vi "ConnectTestDisconnect.vi"() -> ()   [LabVIEW 2019]
panel:
  in  "CircleCenterFinder":bool
  in  "Circle Descriptor":cluster{"Min Radius":dbl, "Max Radius":dbl}={"Min Radius"=50.0, "Max Radius"=80.0}
  out "CircleCenterGH(mm)":string
  out "Image":T1(plugin-control)
  out "NumCirclesFound":i32
  in  "GetHeightGauge Status":bool
  out "HeightGaugeTouch":bool
  out "SDofHeight(mm)":dbl format="%0.3f"
  out "MeanHeight(mm)":dbl format="%0.3f"
  in  "DistSensor":bool
  in  "DropPlate":i32
  out "Position_XYZ":string
  in  "GetGantryXYZ":bool
  in  "DropTool":i32
  in  "PickPlate":u32=50331648
  in  "PickTool":u32=50331648
  in  "Z":dbl=65.0
  in  "PickDrop":bool
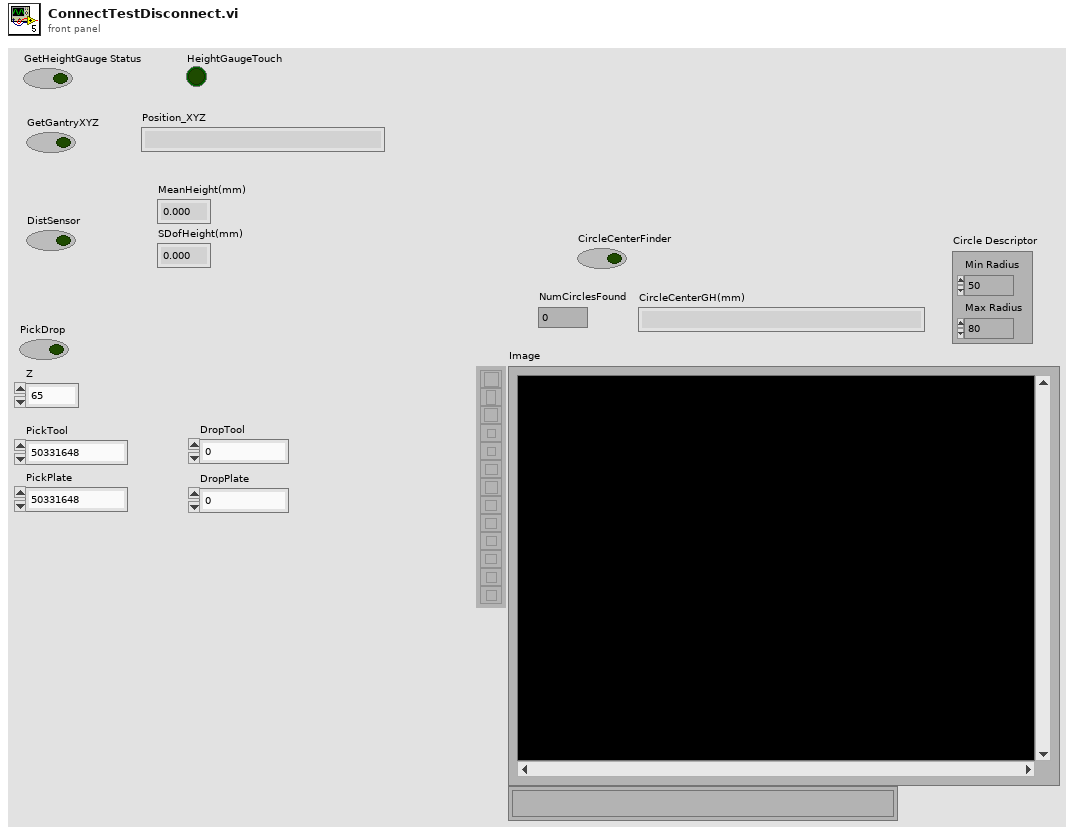
[diagram p1: front panel]
types:
  T1 = typedef "IMAQ Image.ctl" = refnum<image>
  T2 = cluster{"Position":cluster{"X":sgl, "Y":sgl}, "Radius":dbl, "Score":dbl}
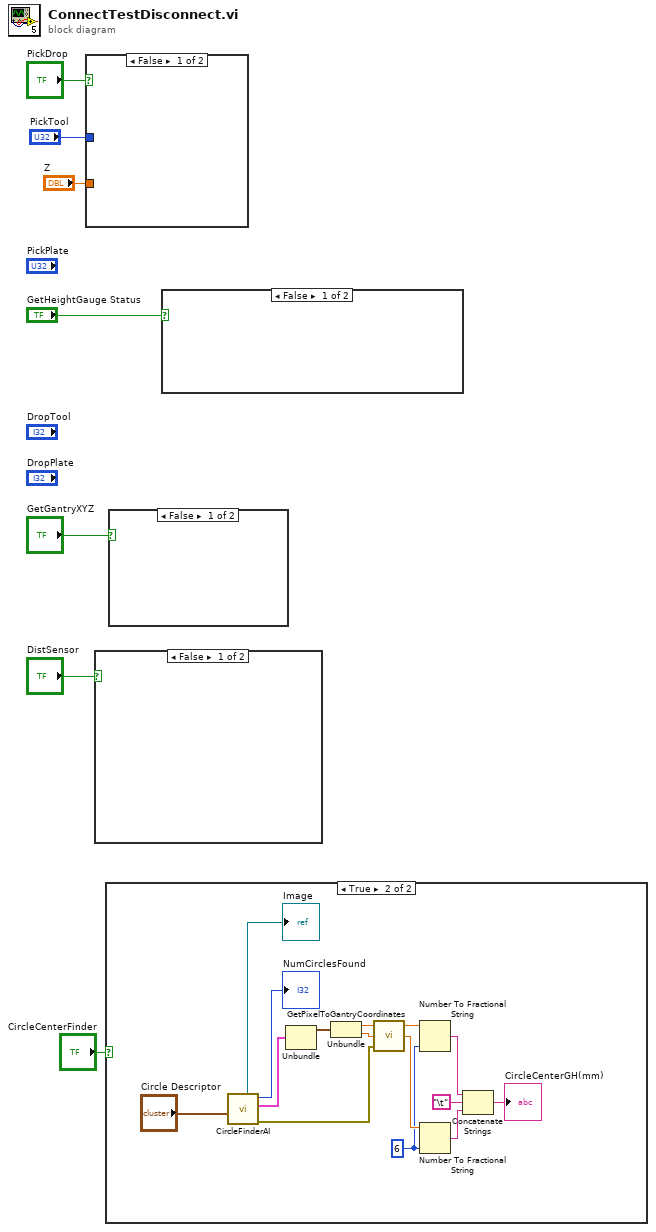
[diagram p0: block diagram]
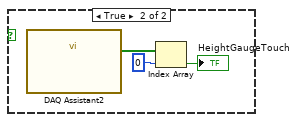
[diagram p3: hidden frame]
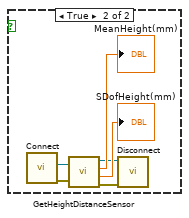
[diagram p4: hidden frame]
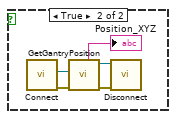
[diagram p5: hidden frame]
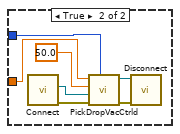
[diagram p6: hidden frame]
diagram:
  n1 = case shown="False" "PickDrop" {
    tunnel: "Z" -> [_ w9]
    tunnel: "PickTool" -> [_ w8]
    frame False {
    }
    frame True {
      n2 = call "Connect.vi"() -> ("error out"=w12:errorcluster, "controller"=w11:refnum<k24>)  [unwired: 10 in]
      n3 = call "PickDropVacCtrld.vi"("VacuumState"=w8, "error in (no error)"=w12, "controller in"=w11, "Zspeed"=50.0, "Z"=w9) -> ("error out"=w13:errorcluster, "controller out"=w14:refnum<k24>)  [unwired: 5 in]
      n4 = call "Disconnect.vi"("error in (no error)"=w13, "controller"=w14) -> ()  [unwired: 9 in, 1 out]
    }
  }
  n5 = case shown="False" "DistSensor" {
    frame False {
    }
    frame True {
      n6 = call "Connect.vi"() -> ("error out"=w16:errorcluster, "controller"=w15:refnum<k24>)  [unwired: 10 in]
      n7 = call "GetHeightDistanceSensor.vi"("controller in"=w15, "error in (no error)"=w16) -> ("controller out"=w17:refnum<k24>, "MeanHeight(mm)"=→"MeanHeight(mm)":dbl, "SDofHeight(mm)"=→"SDofHeight(mm)":dbl, "error out"=w18:errorcluster)
      n8 = call "Disconnect.vi"("error in (no error)"=w18, "controller"=w17) -> ()  [unwired: 9 in, 1 out]
    }
  }
  n9 = case shown="True" "CircleCenterFinder" {
    frame False {
    }
    frame True {
      w26 = i16 6 ("precision (6)")
      n10 = call "CircleFinderAI.vi"("Circle Descriptor"="Circle Descriptor") -> ("error out"=w33:errorcluster, "Circle0"=w32:T2, "NumCirclesFound"=→"NumCirclesFound":i32, "Image"=→"Image":T1)  [unwired: 6 in, 1 out]
      n11 = Unbundle(w32) -> ("Position"=w31:cluster{"X":sgl, "Y":sgl})  [unwired: 2 out]
      n12 = Unbundle(w31) -> ("X"=w30:sgl, "Y"=w29:sgl)
      n13 = call "GetPixelToGantryCoordinates.vi"("error in (no error)"=w33, "PixelY"=w29, "PixelX"=w30) -> ("YmmGH"=w27:dbl, "XmmGH"=w28:dbl)  [unwired: 1 out]
      n14 = Number To Fractional String(number=w28, precision (6)=w26) -> (F-format string=w25:string)  [unwired: 2 in]
      n15 = Number To Fractional String(number=w27, precision (6)=w26) -> (F-format string=w23:string)  [unwired: 2 in]
      n16 = Concatenate Strings(w25, "\t", w23) -> (→"CircleCenterGH(mm)":string)
    }
  }
  n17 = case shown="False" "GetGantryXYZ" {
    frame False {
    }
    frame True {
      n18 = call "Connect.vi"() -> ("error out"=w38:errorcluster, "controller"=w39:refnum<k24>)  [unwired: 10 in]
      n19 = call "GetGantryPosition.vi"("error in (no error)"=w38, "Controller In"=w39) -> ("error out"=w37:errorcluster, "controller out"=w36:refnum<k24>, "Position_XYZ"=→"Position_XYZ":string)  [unwired: 3 in, 4 out]
      n20 = call "Disconnect.vi"("error in (no error)"=w37, "controller"=w36) -> ()  [unwired: 9 in, 1 out]
    }
  }
  n21 = case shown="False" "GetHeightGauge Status" {
    frame False {
    }
    frame True {
      n22 = call "DAQ Assistant2"() -> ("data"=w42:bool[])  [unwired: 17 in, 2 out]
      n23 = Index Array(array=w42, index=0) -> (element=→"HeightGaugeTouch":bool)
    }
  }
